vi "cos_A_cos_a.vi"(1 "AH":dbl, 2 "DEC":dbl, 3 "Latitude Local":dbl) -> (0 "CosAcosa":dbl)   [LabVIEW 2012]
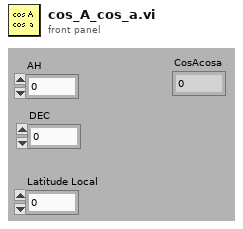
[diagram p1: front panel]
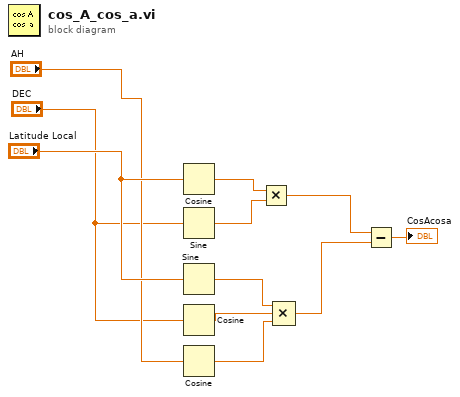
[diagram p0: block diagram]
diagram:
  n1 = Cosine(x="Latitude Local") -> (cos(x)=w4:dbl)
  n2 = Sine(x="DEC") -> (sin(x)=w5:dbl)
  n3 = Sine(x="Latitude Local") -> (sin(x)=w7:dbl)
  n4 = Cosine(x="DEC") -> (cos(x)=w8:dbl)
  n5 = Cosine(x="AH") -> (cos(x)=w9:dbl)
  n6 = Multiply(x=w4, y=w5) -> (x*y=w10:dbl)
  n7 = Compound Arithmetic op=MULTIPLY(w7, w8, w9) -> (w11:dbl)
  n8 = Subtract(x=w10, y=w11) -> (x-y=→"CosAcosa":dbl)
